vi "Read temperature_degC.vi"(8 "error in (no error)":errorcluster, 11 "WSSet in":refnum<class "WSSet.lvclass">) -> (0 "error out":errorcluster, 2 "temperature_degC":dbl[unit]=273.15 min=213.14999999999998 max=333.15, 3 "WSSet out":refnum<class "WSSet.lvclass">)   [LabVIEW 2014, in "TCSDataDefinitions.lvlib" / "TCSWeatherServerCommand.lvlib" / "WSSet.lvclass"]
uses:
  WSSet.lvclass
  WSSet.lvclass/WSSet.ctl
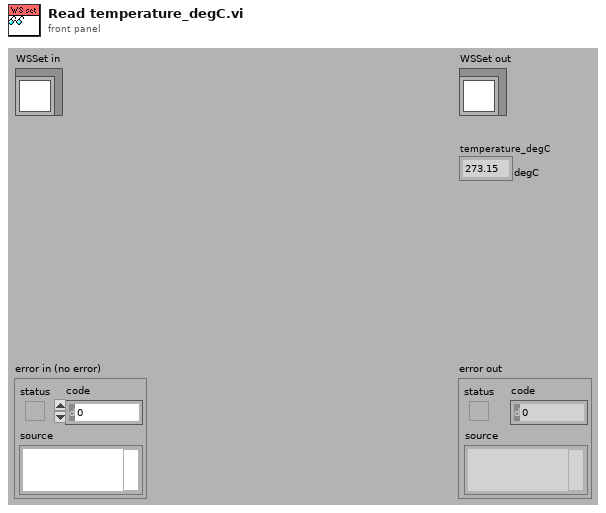
[diagram p1: front panel]
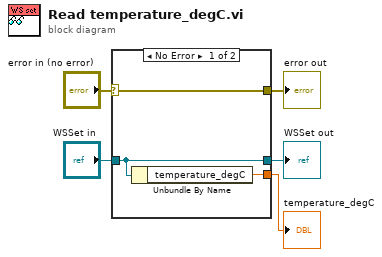
[diagram p0: block diagram]
diagram:
  n1 = case shown="No Error" "error in (no error)" {
    selector: "error in (no error)" -> [w8 w9]
    tunnel: [w8 w9] -> w4
    tunnel: [w7 w10] -> w2
    tunnel: "WSSet in" -> [w7 w10]
    tunnel: [w6 _] -> w1
    frame No Error {
      n2 = Unbundle By Name(w7) -> ("temperature_degC"=w6:dbl[unit])
    }
    frame Error {
    }
  }
  "error out" <- w4
  "WSSet out" <- w2
  "temperature_degC" <- w1
